vi "PustToSyn_RunFinalTest-Standalone.vi"() -> ()   [LabVIEW 2018]
panel:
  in  "File Path":path[](array[path])
  out "result(ary)":string[](array[string])=["Overall Status:  PASS", "Serial Number: RA23070129", "Receive Power Supply Consumption Limits : Pass", "Receiver Input Frequency : Pass", "Receiver Gain : Pass", "Receiver Noise Figure : Pass", "Transmit Output Frequency : Pass", "Transmit Power Supply Consumption Limits : Pass", "Transmit In-Band Output Peak Power : Pass", "Harmonics : Pass", "Reference Source Port Return Loss : Pass", "Transmit Power Flatness : Pass", "Temperature Sensors : Pass", "Bounce Test : Pass"]
  out "Output String":string="REV-C_TETRA_TX-ATTEN database id: 5448\r\nMoved REV-C_TETRA_TX-ATTEN_SN_WAM-000104_2232_060823-120226.csv to Synology Drive\r\nSUCCESS\r\nMoved WAM-C_BOUNCE_SN_WAM-000104_2232_060823-120316_Iq.csv to Synology Drive\r\nWAM-C_BOUNCE database id: 1156\r\nMoved WAM-C_BOUNCE_SN_WAM-000104_2232_060823-120316.csv to Synology Drive\r\nSUCCESS\r\nREV-C_TETRA_TX-PROD-250M database id: 5449\r\nMoved REV-C_TETRA_TX-PROD-250M_SN_WAM-000104_2232_060823-120409.csv to Synology Drive\r\nSUCCESS\r\nCould not move REV-C_TETRA_RX-PROD-250M_SN_WAM-000104_2232_060823-121412_RxCaptureFiles.zip to Synology Drive due to the following error:\r\n[Errno 2] No such file or directory: 'C:\\\\RageATE Results\\\\REV-C_TETRA_RX-PROD-250M\\\\6_8_2023\\\\REV-C_TETRA_RX-PROD-250M_SN_WAM-000104_2232_060823-121412_RxCaptureFiles.zip'\r\nREV-C_TETRA_RX-PROD-250M database id: 5450\r\nMoved REV-C_TETRA_RX-PROD-250M_SN_WAM-000104_2232_060823-121412.csv to Synology Drive\r\nSUCCESS"
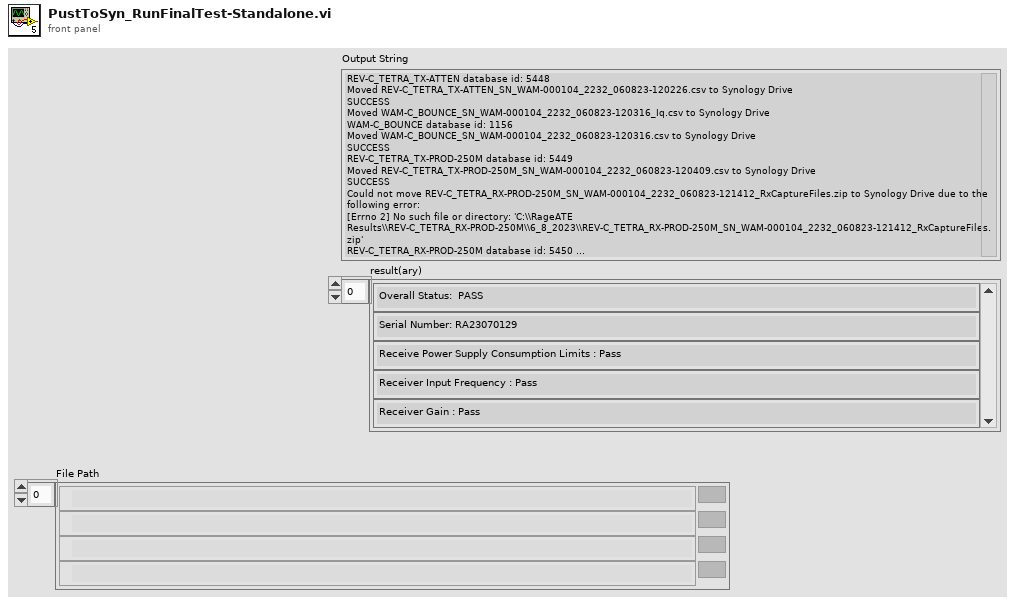
[diagram p1: front panel]
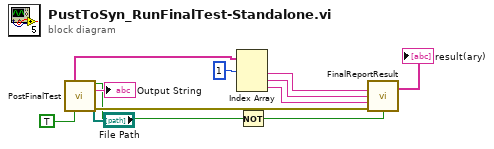
[diagram p0: block diagram]
diagram:
  n1 = call "PostFinalTest.vi"("File Path"="File Path", "Enable(t)"=TRUE) -> ("ID"=w11:string[], "error?(t)"=w3:bool, "Output String"=→"Output String":string, "error out"=w12:errorcluster)  [unwired: 8 in, 2 out]
  n2 = Index Array(array=w11, index #1=1 ("index")) -> (element #1=w7:string, element #2=w9:string, element #3=w10:string)  [unwired: 2 in]
  n3 = Not(x=w3) -> (.not. x?=w2:bool)
  n4 = call "FinalReportResult.vi"("TXID"=w7, "RXID"=w9, "BOUNCEID"=w10, "error in (no error)"=w12, "Run Final Report (T)"=w2) -> ("result(ary)"=→"result(ary)":string[])  [unwired: 6 in, 4 out]
